vi "Analog Voltage Read.vi"(4 "samples per channel":i32=1000, 6 "rate":dbl=1000.0 format="%0.2f", 8 "sample mode":i32(ring)=10178 items=["Finite Samples"=10178, "Continuous Samples"=10123, "Hardware Timed Single Point"=12522], 9 "maximum value":dbl=5.0 format="%0.2f", 10 "minimum value":dbl=-5.0 format="%0.2f", 11 "physical channels":tag) -> (2 "data":dbl)   [LabVIEW 2014]
uses:
  <vilib>/Utility/error.llb/DialogType.ctl
  <vilib>/DAQmx/read.llb/DAQmx Read (Analog DBL 1Chan 1Samp).vi
  <vilib>/DAQmx/create/channels.llb/DAQmx Create Channel (AI-Voltage-Basic).vi
  <vilib>/DAQmx/configure/timing.llb/DAQmx Timing (Sample Clock).vi
  <vilib>/DAQmx/miscellaneous.llb/DAQmx Fill In Error Info.vi
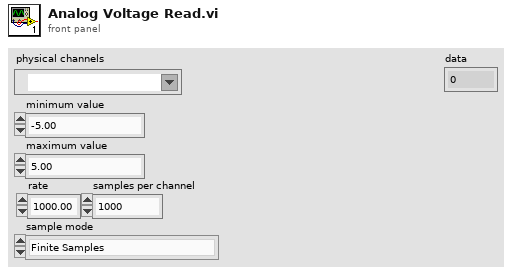
[diagram p1: front panel]
types:
  T1 = typedef "DialogType.ctl" = u16
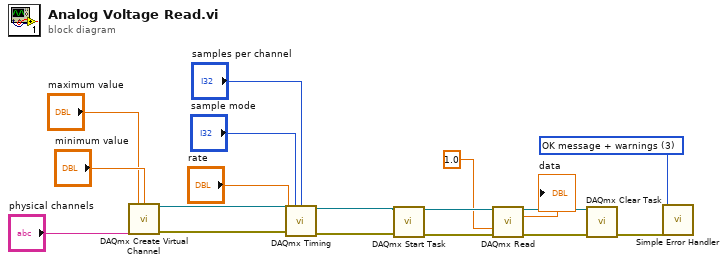
[diagram p0: block diagram]
diagram:
  w3 = T1 3 items=["no dialog", "OK message", "continue or stop message", "OK message + warnings", "continue/stop + warnings"] ("type of dialog (OK msg:1)")
  n1 = call-poly <vilib>:"DAQmx Create Virtual Channel.vi"("maximum value"="maximum value", "minimum value"="minimum value", "physical channels"="physical channels") -> ("task out"=w15:refnum<k21>, "error out"=w14:errorcluster)  [unwired: 11 in]
  n2 = call-poly <vilib>:"DAQmx Timing.vi"("task/channels in"=w15, "sample mode"="sample mode", "samples per channel"="samples per channel", "rate"="rate", "error in"=w14) -> ("task out"=w11:refnum<k21>, "error out"=w10:errorcluster)  [unwired: 9 in]
  n3 = call <vilib>:"DAQmx Start Task.vi"("task/channels in"=w11, "error in"=w10) -> ("task out"=w9:refnum<k21>, "error out"=w8:errorcluster)  [unwired: 12 in]
  n4 = call-poly <vilib>:"DAQmx Read.vi"("task/channels in"=w9, "timeout"=1.0, "error in"=w8) -> ("task out"=w6:refnum<k21>, "data"=→"data":dbl, "error out"=w5:errorcluster)  [unwired: 10 in]
  n5 = call <vilib>:"DAQmx Clear Task.vi"("task in"=w6, "error in"=w5) -> ("error out"=w4:errorcluster)  [unwired: 13 in]
  n6 = call <vilib>:"Simple Error Handler.vi"("type of dialog (OK msg:1)"=w3, "error in (no error)"=w4) -> ()  [unwired: 3 in, 5 out]
